vi "setTraceVisib.vi"(6 "showAll array 2":refnum<vi>[](array[refnum]), 8 "show3 array 3":refnum<vi>[](array[refnum]), 9 "NewVal":enum32{"All", "3Channels"}(ring), 10 "All Channel":refnum<vi>, 11 "wavegaph array 2":refnum<vi>[](array[refnum])) -> ()   [LabVIEW 2013]
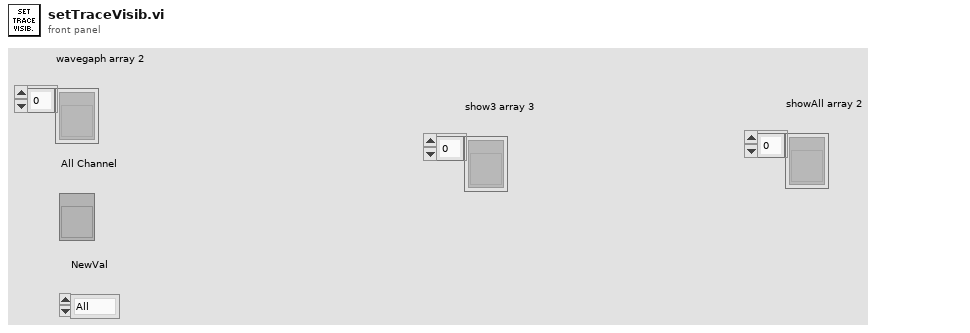
[diagram p1: front panel]
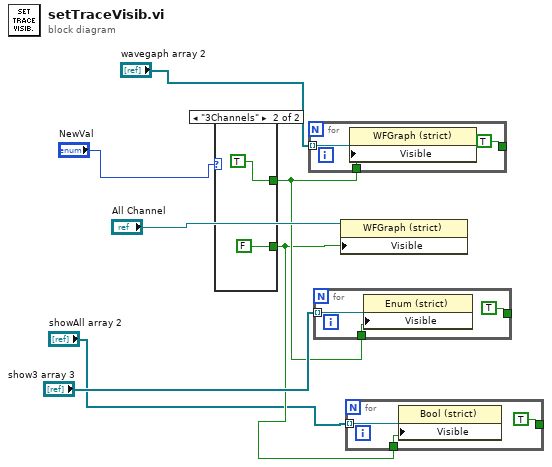
[diagram p0: block diagram]
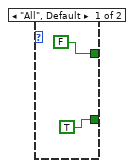
[diagram p2: hidden frame]
diagram:
  n1 = case shown="\"3Channels\"" "NewVal" {
    tunnel: [TRUE ("Visible") FALSE ("Visible")] -> w2
    tunnel: [FALSE ("Visible") TRUE ("Visible")] -> w3
    frame "All", Default {
    }
    frame "3Channels" {
    }
  }
  n2 = for {
    tunnel: "wavegaph array 2" -> [w14] mode=indexing
    tunnel: [TRUE] -> _
    tunnel: w3 -> [w12]
    n3 = property class="WFGraph (strict)"(reference=w14, "Visible"=w12) -> ()  [unwired: 1 in, 2 out]
  }
  n4 = for {
    tunnel: "show3 array 3" -> [w17] mode=indexing
    tunnel: [TRUE] -> _
    tunnel: w3 -> [w15]
    n5 = property class="Enum (strict)"(reference=w17, "Visible"=w15) -> ()  [unwired: 1 in, 2 out]
  }
  n6 = property class="WFGraph (strict)"(reference="All Channel", "Visible"=w2) -> ()  [unwired: 1 in, 2 out]
  n7 = for {
    tunnel: "showAll array 2" -> [w20] mode=indexing
    tunnel: [TRUE] -> _
    tunnel: w2 -> [w18]
    n8 = property class="Bool (strict)"(reference=w20, "Visible"=w18) -> ()  [unwired: 1 in, 2 out]
  }
